vi "Set Frame Channel.vi"(8 "error in (no error)":errorcluster, 9 "channel":i32, 10 "frame":i32, 11 "Chroma190020 HiPOT in":refnum<class "Chroma190020 HiPOT.lvclass">) -> (0 "error out":errorcluster, 3 "Chroma190020 HiPOT out":refnum<class "Chroma190020 HiPOT.lvclass">)   [LabVIEW 2019, in "Concrete.lvlib" / "Chroma190020 HiPOT.lvclass"]
uses:
  Chroma190020 HiPOT.lvclass
  Chroma190020 HiPOT.lvclass/Chroma190020 HiPOT.ctl
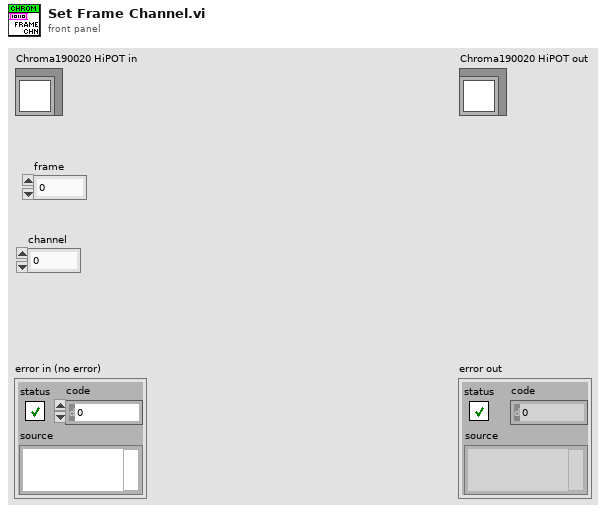
[diagram p1: front panel]
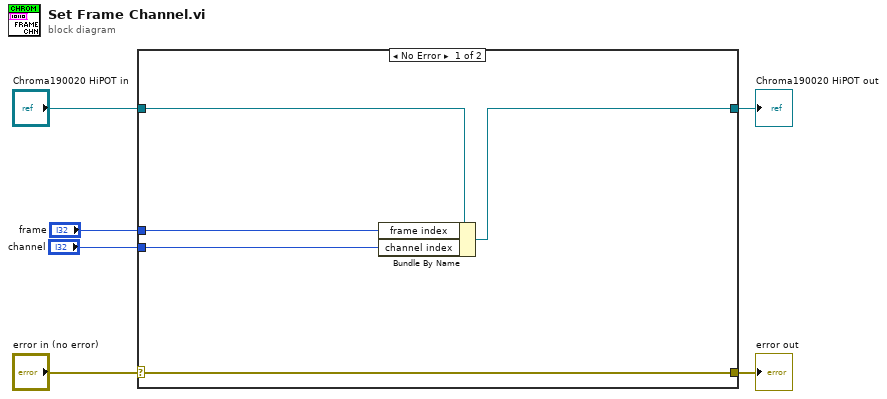
[diagram p0: block diagram]
diagram:
  n1 = case shown="No Error" "error in (no error)" {
    selector: "error in (no error)" -> [w11 w13]
    tunnel: [w11 w13] -> w5
    tunnel: [w9 w12] -> w3
    tunnel: "Chroma190020 HiPOT in" -> [w10 w12]
    tunnel: "frame" -> [w8 _]
    tunnel: "channel" -> [w7 _]
    frame No Error {
      n2 = Bundle By Name(cluster=w10, "frame index"=w8, "channel index"=w7) -> (w9:refnum<class "Chroma190020 HiPOT.lvclass">)
    }
    frame Error {
    }
  }
  "error out" <- w5
  "Chroma190020 HiPOT out" <- w3
